vi "NormalizeSignalTiming.vi"(11 "Input Signals":T1[](array[typedef])) -> (3 "Aligned Signals":T1[](array[typedef]))   [LabVIEW 2016]
uses:
  Ctrl_Signal.ctl
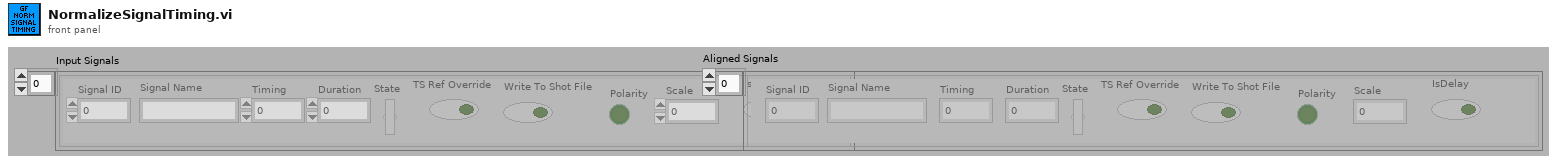
[diagram p1: front panel]
types:
  T1 = typedef "Ctrl_Signal.ctl" = cluster{"Signal Name":string, "Timing":dbl, "Duration":dbl, "State":bool, "TS Ref Override":bool, "Write To Shot File":bool, "Polarity":bool, "Signal ID":dbl, "Scale":dbl, "IsDelay":bool}
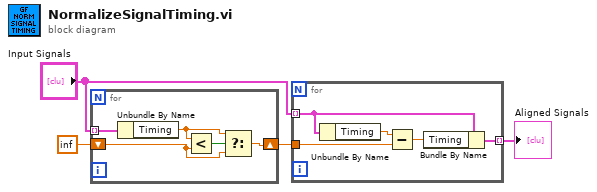
[diagram p0: block diagram]
diagram:
  n1 = for {
    tunnel: "Input Signals" -> [w9] mode=indexing
    shift-right: [w5] -> w1
    shift-left: inf -> [w6]
    n2 = Unbundle By Name(w9) -> ("Timing"=w7:dbl)
    n3 = Less?(x=w7, y=w6) -> (x < y?=w8:bool)
    n4 = Select(t=w7, s=w8, f=w6) -> (s? t:f=w5:dbl)
  }
  n5 = for {
    tunnel: [w14] -> w3 mode=indexing
    tunnel: "Input Signals" -> [w13] mode=indexing
    tunnel: w1 -> [w10]
    n6 = Unbundle By Name(w13) -> ("Timing"=w12:dbl)
    n7 = Subtract(x=w12, y=w10) -> (x-y=w11:dbl)
    n8 = Bundle By Name(cluster=w13, "Timing"=w11) -> (w14:T1)
  }
  "Aligned Signals" <- w3
